vi "Get UTF Status.vi"(8 "Error In":errorcluster, 11 "UTF Results":T2) -> (0 "Error Out":errorcluster, 2 "Status":T1=enum."Passed", 3 "UTF Results":T2)   [LabVIEW 2013, in "VIChallenge.lvlib"]
uses:
  VIChallenge.lvlib
  <vilib>/utf/common/utf_test_result_overall.ctl
  <vilib>/utf/common/utf_test_result_testfile.ctl
  <vilib>/utf/common/utf_test_result_testcase.ctl
  <vilib>/utf/common/utf_test_result.ctl
  <vilib>/utf/common/utf_test_result_troll_new.ctl
  <vilib>/utf/common/utf_vector_result.ctl
  <vilib>/utf/common/utf_test_result_failure.ctl
  <vilib>/utf/common/utf_test_comparison_operators.ctl
  <vilib>/utf/common/utf_vi_tag.ctl
  <vilib>/utf/common/utf_test_result_input_data.ctl
  <vilib>/utf/common/utf_code_coverage.ctl
  <vilib>/utf/common/utf_error_data.ctl
  <vilib>/utf/common/utf_error_type.ctl
  <vilib>/utf/common/utf_subvi_info.ctl
  Type Defs/UTF Status.ctl
  <vilib>/utf/NI_UnitTestFramework.lvlib
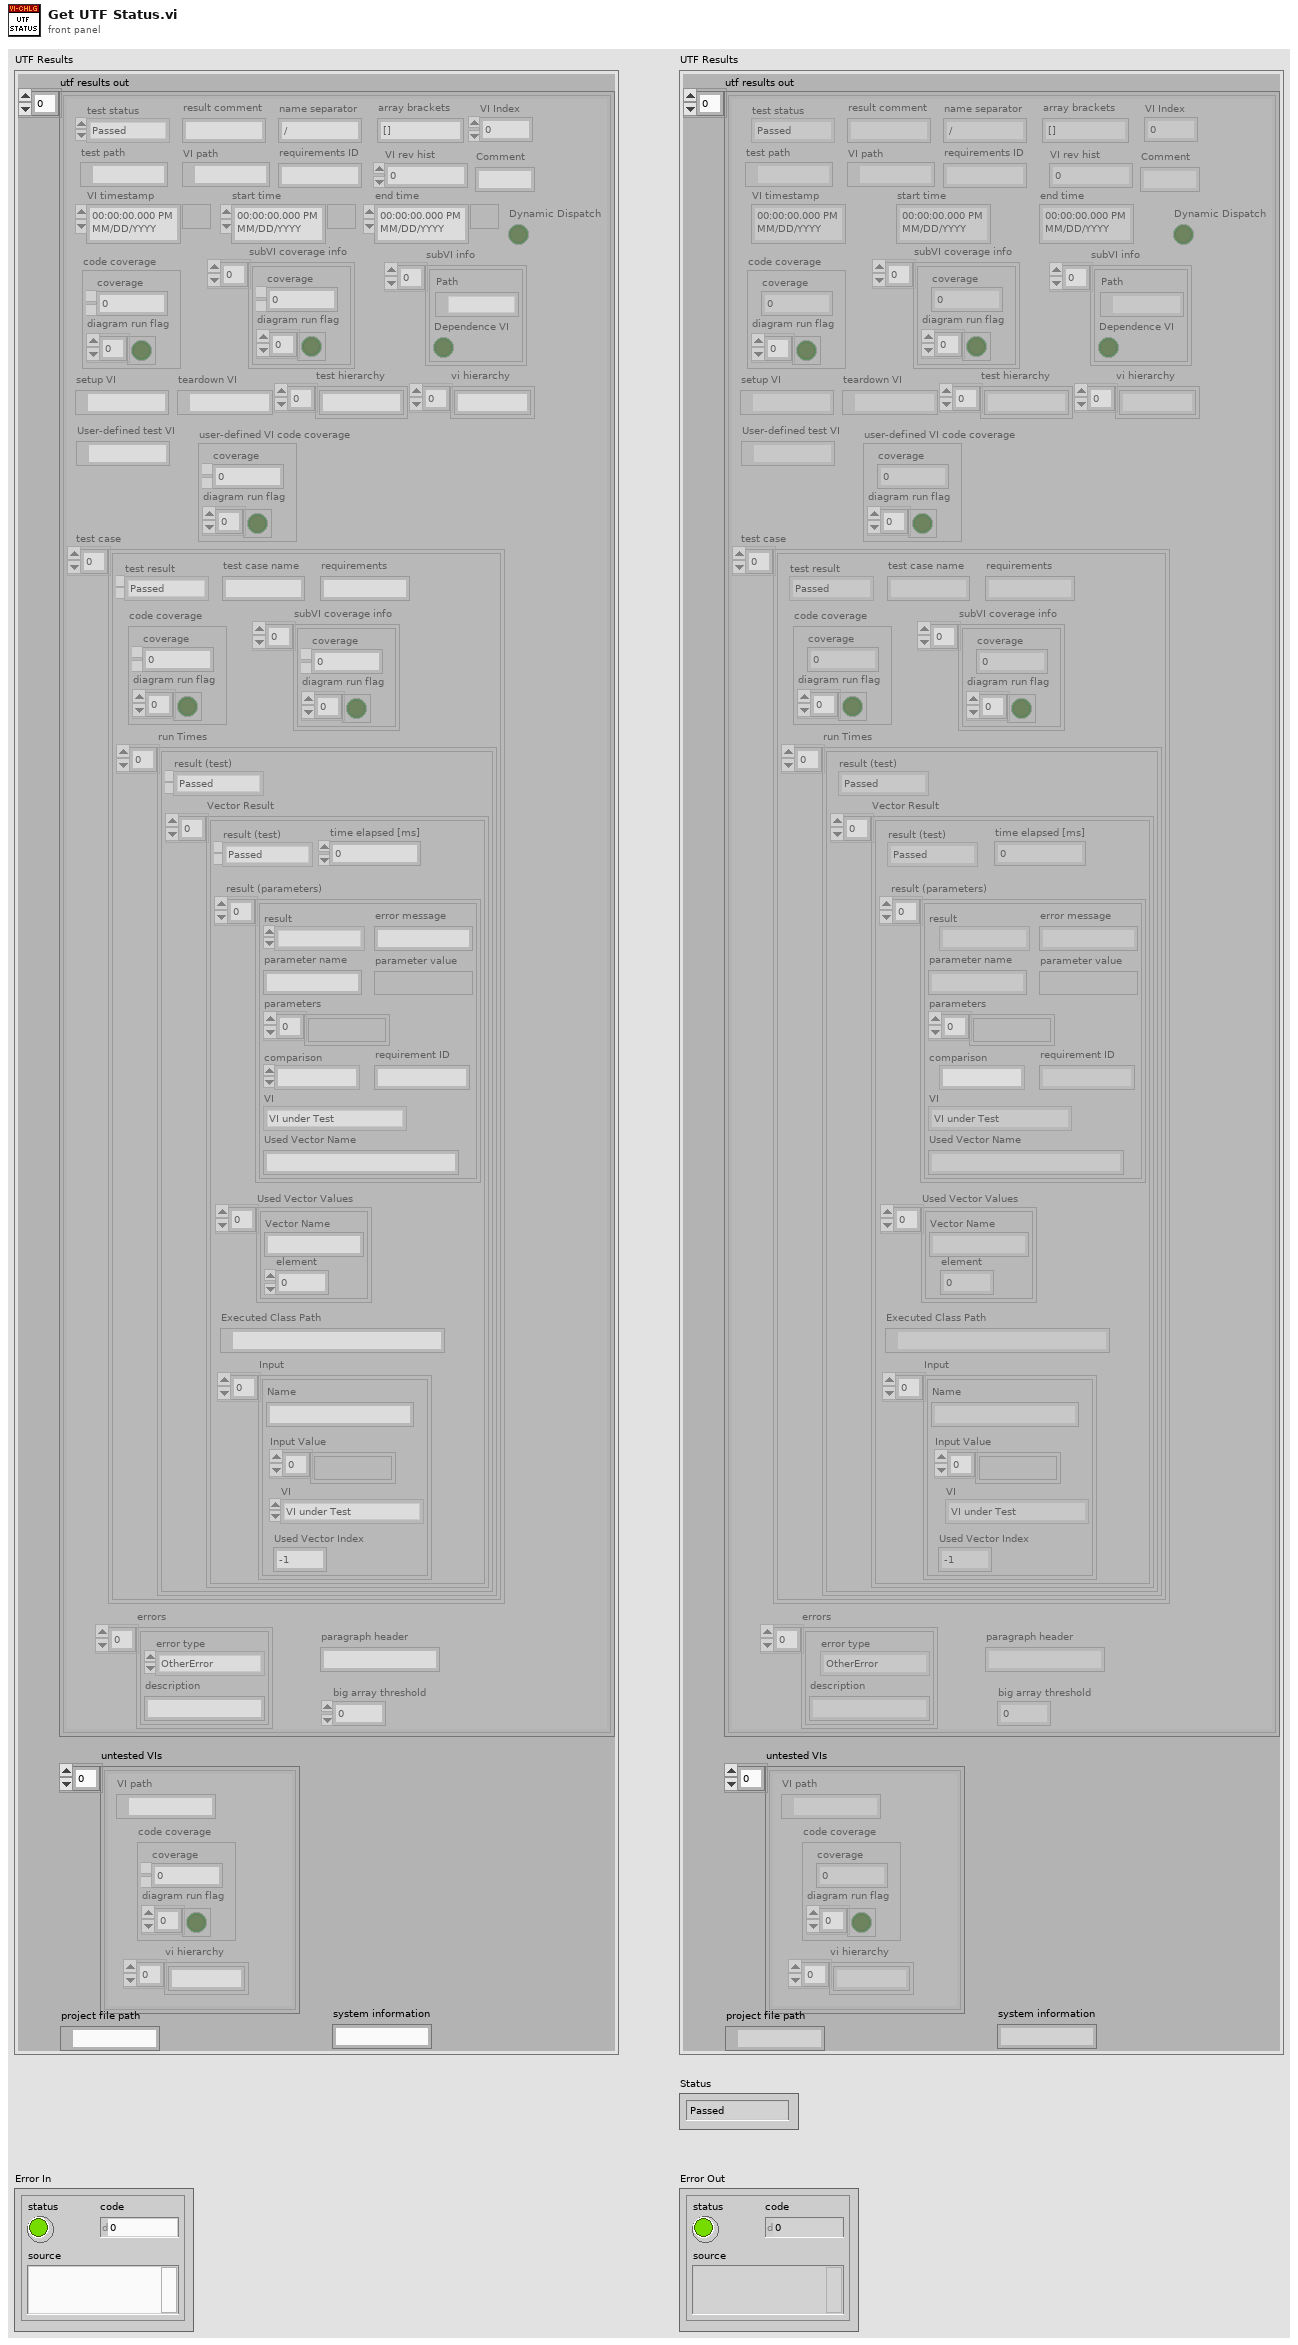
[diagram p1: front panel]
types:
  T1 = typedef "VIChallenge.lvlib/UTF Status.ctl" = enum16{"Null", "Passed", "Failed", "Error", "Skipped", "Not Processed"}
  T2 = typedef "NI_UnitTestFramework.lvlib/utf_test_result_overall.ctl" = cluster{"utf results out":T3[], "untested VIs":cluster{"VI path":path, "code coverage":T12, "vi hierarchy":string[]}[], "project file path":path, "system information":string}
  T3 = typedef "NI_UnitTestFramework.lvlib/utf_test_result_testfile.ctl" = cluster{"test case":T4[], "test status":T5, "test path":path, "setup VI":path, "teardown VI":path, "code coverage":T12, "start time":timestamp, "end time":timestamp, "test hierarchy":string[], "VI path":path, "VI timestamp":timestamp, "VI rev hist":i32, "requirements ID":string, "array brackets":string, "name separator":string, "errors":T13[], "paragraph header":string, "result comment":string, "vi hierarchy":string[], "subVI coverage info":T12[], "subVI info":T15[], "big array threshold":u32, "VI Index":i32, "Comment":string, "Dynamic Dispatch":bool, "User-defined test VI":path, "user-defined VI code coverage":T12}
  T4 = typedef "NI_UnitTestFramework.lvlib/utf_test_result_testcase.ctl" = cluster{"test result":T5, "run Times":T6[], "test case name":string, "requirements":string, "code coverage":T12, "subVI coverage info":T12[]}
  T5 = typedef "NI_UnitTestFramework.lvlib/utf_test_result.ctl" = enum16{"Passed", "Failed", "Error", "Skipped", "Not Processed"}
  T6 = typedef "NI_UnitTestFramework.lvlib/utf_test_result_troll_new.ctl" = cluster{"result (test)":T5, "Vector Result":T7[]}
  T7 = typedef "NI_UnitTestFramework.lvlib/utf_vector_result.ctl" = cluster{"time elapsed [ms]":u32, "result (test)":T5, "result (parameters)":T8[], "Used Vector Values":cluster{"Vector Name":string, "element":i32}[], "Executed Class Path":path, "Input":T11[]}
  T8 = typedef "NI_UnitTestFramework.lvlib/utf_test_result_failure.ctl" = cluster{"result":T5, "error message":string, "parameter name":string, "parameter value":variant, "parameters":variant[], "comparison":T9, "requirement ID":string, "VI":T10, "Used Vector Name":string}
  T9 = typedef "NI_UnitTestFramework.lvlib/utf_test_comparison_operators.ctl" = enum16{"=", "!=", ">", ">=", "<", "<=", "range", "symmetric tolerance", "asymmetric tolerance", "string contains", "string not contain", "array size", "string length", "array range", "by element", "array range (limit array)", "user-defined", "array contains", "array not contain", "vector length", "= (elm)", "!= (elm)", "= (case insensitive)", "!= (case insensitive)"}
  T10 = typedef "NI_UnitTestFramework.lvlib/utf_vi_tag.ctl" = enum16{"Setup VI", "VI under Test", "Teardown VI"}
  T11 = typedef "NI_UnitTestFramework.lvlib/utf_test_result_input_data.ctl" = cluster{"Name":string, "Input Value":variant[], "VI":T10, "Used Vector Index":i32}
  T12 = typedef "NI_UnitTestFramework.lvlib/utf_code_coverage.ctl" = cluster{"coverage":dbl, "diagram run flag":bool[]}
  T13 = typedef "NI_UnitTestFramework.lvlib/utf_error_data.ctl" = cluster{"error type":T14, "description":string}
  T14 = typedef "NI_UnitTestFramework.lvlib/utf_error_type.ctl" = enum16{"TestFileError", "VIError", "SetupVIError", "TearDownVIError", "OtherError"}
  T15 = typedef "NI_UnitTestFramework.lvlib/utf_subvi_info.ctl" = cluster{"Path":path, "Dependence VI":bool}
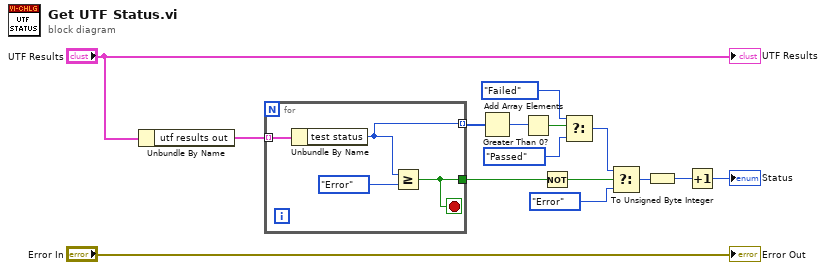
[diagram p0: block diagram]
diagram:
  n1 = Unbundle By Name("UTF Results") -> ("utf results out"=w14:T3[])
  n2 = for {
    tunnel: w14 -> [w19] mode=indexing
    tunnel: [w17] -> w7
    tunnel: [w16] -> w12 mode=indexing
    stop <- w17 stop-if-true
    n3 = Unbundle By Name(w19) -> ("test status"=w16:T5)
    n4 = Greater Or Equal?(x=w16, y=utf_test_result."Error") -> (x >= y?=w17:bool)
  }
  n5 = Add Array Elements(numeric array=w12) -> (sum=w11:T5)
  n6 = Greater Than 0?(x=w11) -> (x > 0?=w10:bool)
  n7 = Not(x=w7) -> (.not. x?=w6:bool)
  n8 = Select(t=utf_test_result."Failed" ("y"), s=w10, f=utf_test_result."Passed" ("y")) -> (s? t:f=w5:T5)
  n9 = Select(t=w5, s=w6, f=utf_test_result."Error" ("y")) -> (s? t:f=w3:T5)
  n10 = To Unsigned Byte Integer(number=w3) -> (unsigned 8bit integer=w2:u8)
  n11 = Increment(x=w2) -> (x+1=→"Status":u8)
  "Error Out" <- "Error In"
  "UTF Results" <- "UTF Results"
